vi "Read Value.vi"(8 "error in (no error)":errorcluster, 11 "Output Channels in":refnum<class "Output Channels.lvclass">) -> (0 "error out":errorcluster, 2 "Value":dbl, 3 "Output Channels out":refnum<class "Output Channels.lvclass">)   [LabVIEW 2020, in "Plugin.lvlib" / "Output Channels.lvclass"]
doc: "Read Value"
uses:
  Output Channels.lvclass
  Output Channels.lvclass/Output Channels.ctl
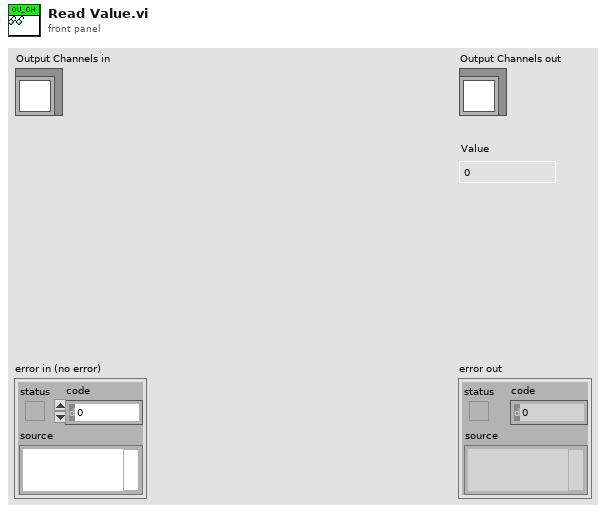
[diagram p1: front panel]
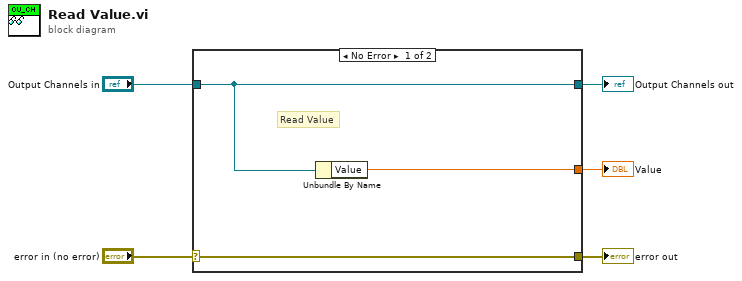
[diagram p0: block diagram]
diagram:
  n1 = case shown="No Error" "error in (no error)" {
    selector: "error in (no error)" -> [w8 w9]
    tunnel: [w8 w9] -> w4
    tunnel: [w7 w10] -> w2
    tunnel: "Output Channels in" -> [w7 w10]
    tunnel: [w6 _] -> w1
    frame No Error {
      # "Read Value"
      n2 = Unbundle By Name(w7) -> ("Value"=w6:dbl)
    }
    frame Error {
    }
  }
  "error out" <- w4
  "Output Channels out" <- w2
  "Value" <- w1
